vi "Events to Listbox.vi"(8 "error in":errorcluster, 10 "Events":T1[](array[typedef]), 11 "Listbox ref":refnum<vi>) -> (0 "error out":errorcluster, 3 "Listbox ref out":refnum<vi>)   [LabVIEW 2020]
uses:
  Utilities/iCalendar/Extract iCalendar String.ctl
panel:
  out "Listbox out":i32(listbox)
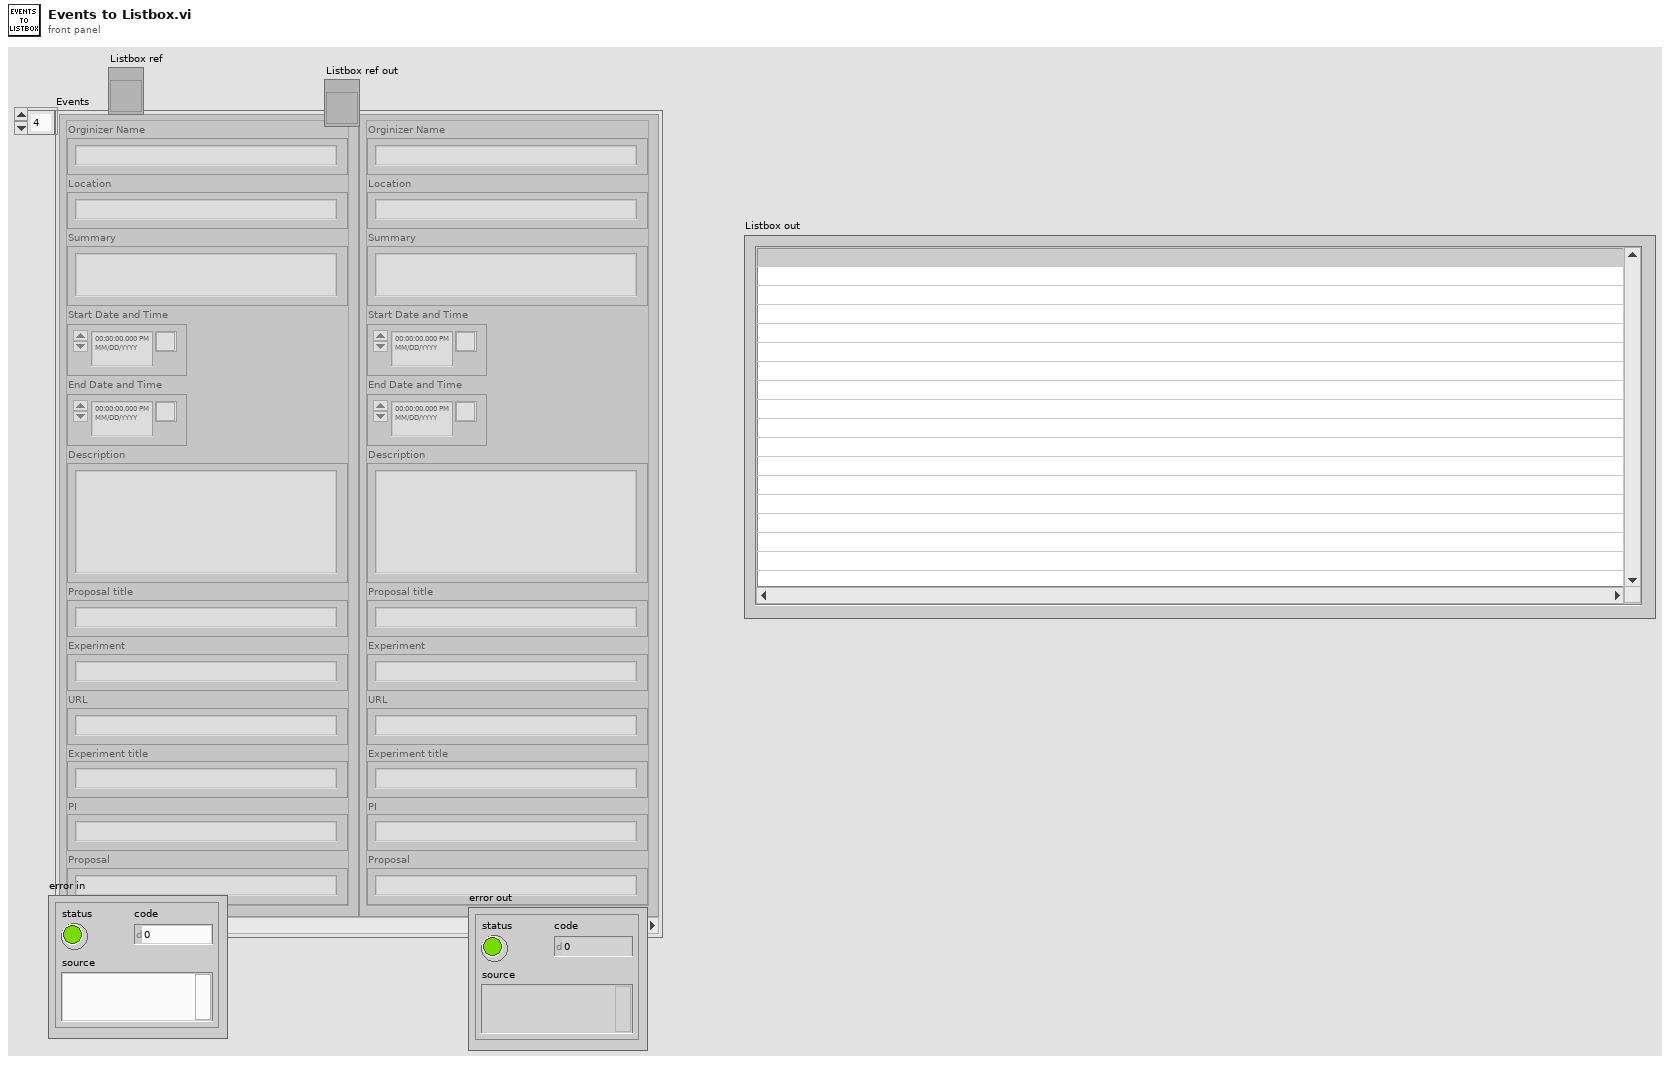
[diagram p1: front panel]
types:
  T1 = typedef "Extract iCalendar String.ctl" = cluster{"Orginizer Name":string, "Location":string, "Summary":string, "Start Date and Time":timestamp, "End Date and Time":timestamp, "Description":string, "Proposal title":string, "Experiment":string, "URL":string, "Experiment title":string, "PI":string, "Proposal":string}
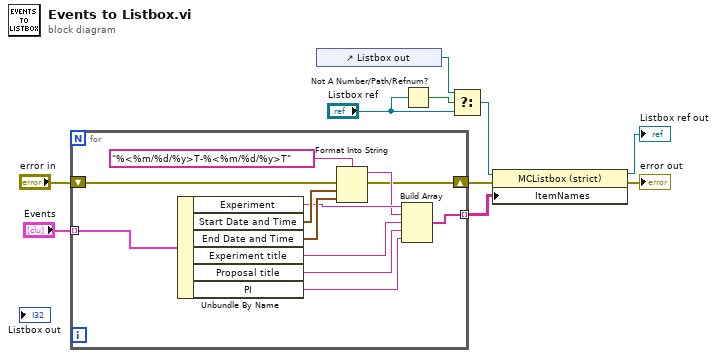
[diagram p0: block diagram]
diagram:
  n1 = for {
    tunnel: "Events" -> [w22] mode=indexing
    shift-right: [w14] -> w6
    shift-left: "error in" -> [w15]
    tunnel: [w13] -> w5 mode=indexing
    n2 = Unbundle By Name(w22) -> ("Experiment"=w18:string, "Start Date and Time"=w20:timestamp, "End Date and Time"=w19:timestamp, "Experiment title"=w12:string, "Proposal title"=w17:string, "PI"=w11:string)
    n3 = Format Into String(format string="%<%m/%d/%y>T-%<%m/%d/%y>T", error in=w15, w20, w19) -> (resulting string=w16:string, error out=w14:errorcluster)  [unwired: 1 in]
    n4 = Build Array(w18, w16, w12, w17, w11) -> (w13:string[])
  }
  n5 = control-ref of="Listbox out"() -> (w3:refnum<vi>)
  n6 = Not A Number/Path/Refnum?(number/path/refnum="Listbox ref") -> (NaN/Path/Refnum?=w4:bool)
  n7 = Select(t=w3, s=w4, f="Listbox ref") -> (s? t:f=w1:refnum<vi>)
  n8 = property class="MCListbox (strict)"(reference=w1, error in=w6, "ItemNames"=w5) -> (reference out=→"Listbox ref out":refnum<vi>, error out=→"error out":errorcluster)
